vi "Prepare FTP Files.vi"(11 "file (use dialog)":path) -> (1 "MPUT Refnum out":refnum<file>, 2 "MGET Refnum out":refnum<file>)   [LabVIEW 2014]
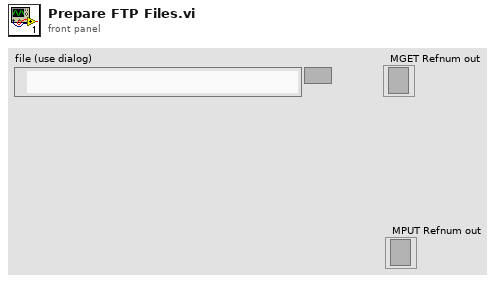
[diagram p1: front panel]
types:
  T1 = enum16{"open", "replace", "create", "open or create", "replace or create", "replace or create with confirmation"}
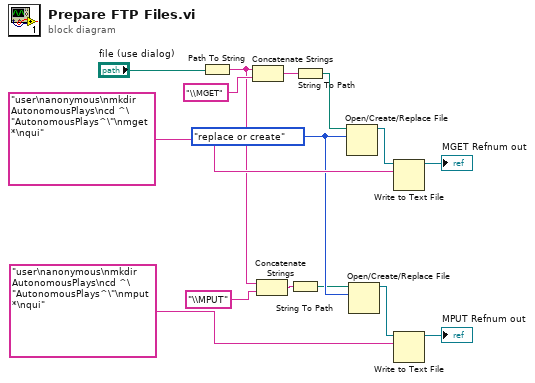
[diagram p0: block diagram]
diagram:
  w10 = T1."replace or create" ("operation (0:open)")
  n1 = Path To String(path="file (use dialog)") -> (string=w3:string)
  n2 = Concatenate Strings(w3, "\\MGET" ("string")) -> (w7:string)
  n3 = Concatenate Strings(w3, "\\MPUT" ("string")) -> (w1:string)
  n4 = String To Path(string=w1) -> (path=w2:path)
  n5 = String To Path(string=w7) -> (path=w5:path)
  n6 = Open/Create/Replace File(file path (use dialog)=w5, operation (0:open)=w10) -> (refnum out=w11:refnum<file>)  [unwired: 4 in, 2 out]
  n7 = Open/Create/Replace File(file path (use dialog)=w2, operation (0:open)=w10) -> (refnum out=w9:refnum<file>)  [unwired: 4 in, 2 out]
  n8 = Write to Text File(file (use dialog)=w11, text="user\nanonymous\nmkdir AutonomousPlays\ncd ^\"AutonomousPlays^\"\nmget *\nqui") -> (refnum out=→"MGET Refnum out":refnum<file>)  [unwired: 2 in, 2 out]
  n9 = Write to Text File(file (use dialog)=w9, text="user\nanonymous\nmkdir AutonomousPlays\ncd ^\"AutonomousPlays^\"\nmput *\nqui") -> (refnum out=→"MPUT Refnum out":refnum<file>)  [unwired: 2 in, 2 out]
